vi "dynamatic.vi"(8 "error in (no error)":errorcluster, 11 "CParent in":refnum<class "CParent.lvclass">) -> (0 "error out":errorcluster, 2 "String":string, 3 "CParent out":refnum<class "CParent.lvclass">)   [LabVIEW 2024, in "CParent.lvclass"]
uses:
  CParent.lvclass
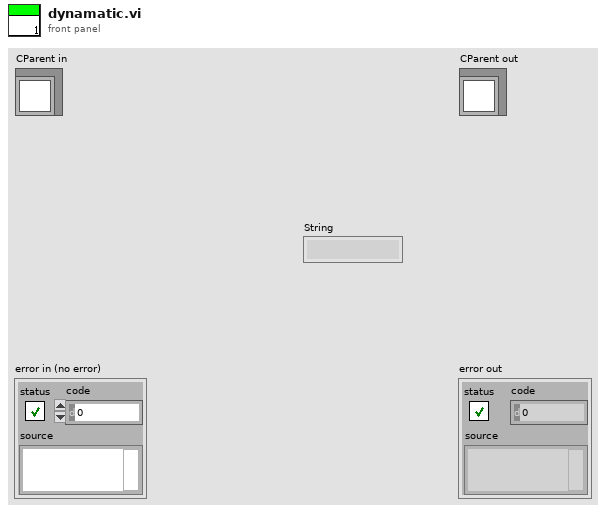
[diagram p1: front panel]
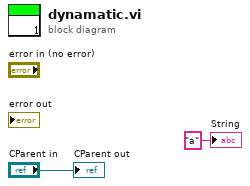
[diagram p0: block diagram]
diagram:
  "CParent out" <- "CParent in"
  "String" <- "a" ("String")
